vi "emballage mise en forme pour commandes en cours.vi"(2 "Nb pièces emballées":u64=28, 3 "pièces emballées":string[][](array[string])=[["12-216E_01_25 F120023 500mA 10ohm", "501356760408101040", "25.03.2008 10:52", "MQI", "10407/06-01.31.03", "2", "50"], ["12-216E_01_25 F120023 500mA 10ohm", "501356760408101040", "25.03.2008 10:53", "MQI", "10407/06-01.31.03", "1", "50"]]) -> (0 "Chaîne pour fichier cmde":string="12-216E_01_25 F120023 500mA 10ohm\t25.03.2008 10:52\tMQI\t10407/06-01.31.03\t2\t28/50")   [LabVIEW 2020]
panel:
  # "nom valve"
  # "n° code bar"
  # "nom OP"
  # "n°cmde"
  # "n° carton"
  # "qtté TOT à emballer"
  # "date+heure"
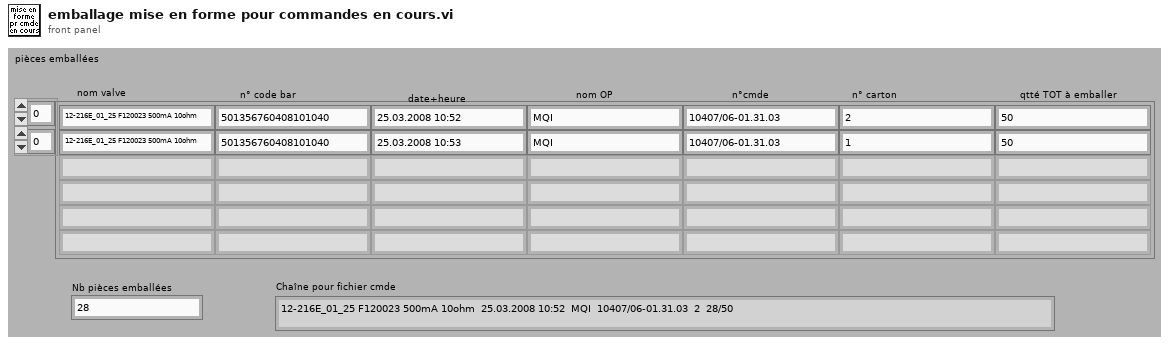
[diagram p1: front panel]
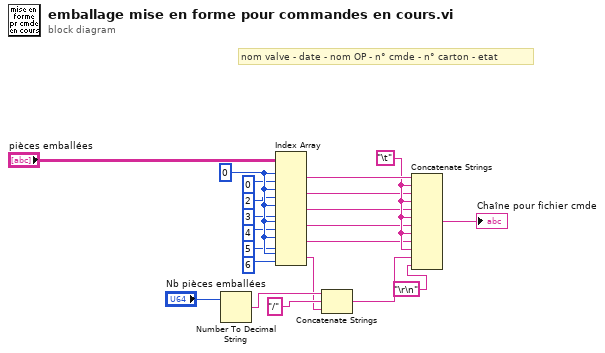
[diagram p0: block diagram]
diagram:
  w12 = "\t"
  w20 = 0
  # "nom valve - date - nom OP - n° cmde - n° carton - etat"
  n1 = Number To Decimal String(number="Nb pièces emballées") -> (decimal integer string=w10:string)  [unwired: 1 in]
  n2 = Index Array(array="pièces emballées", index (row) #1=w20, index (col) #1=0, index (row) #2=w20, index (col) #2=2, index (row) #3=w20, index (col) #3=3, index (row) #4=w20, index (col) #4=4, index (row) #5=w20, index (col) #5=5, index (row) #6=w20, index (col) #6=6) -> (element #1=w13:string, element #2=w7:string, element #3=w6:string, element #4=w5:string, element #5=w4:string, element #6=w3:string)
  n3 = Concatenate Strings(w10, "/", w3) -> (w8:string)
  n4 = Concatenate Strings(w13, w12, w7, w12, w6, w12, w5, w12, w4, w12, w8, "\r\n") -> (→"Chaîne pour fichier cmde":string)
